vi "Ramp.vi"(8 "Control":u32, 9 "Switch 2":bool, 10 "Switch 1":bool) -> ()   [LabVIEW 2018]
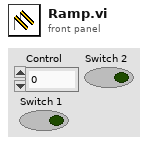
[diagram p1: front panel]
types:
  T1 = typedef "WPI_MotorControlDeviceRef.ctl" = cluster{"DeviceStatus":errorcluster, "Type":T2, "PWM":cluster{"PWM Channel":T3, "DeadBand":T4}, "CAN":cluster{"Device Number":u8, "SetOutput VI Ref":variant, "GetOutput VI Ref":variant, "Enable VI Ref":variant, "Disable VI Ref":variant, "Data":variant}, "Invert":bool, "DIO PWM":cluster{"PWM \"Enable\" Channel":T3, "DIOChannel":T5, "PWM Rate":dbl}}
  T2 = typedef "WPI_MotorControlType.ctl" = enum16{"PWM", "CAN", "DIO PWM"}
  T3 = typedef "FPGA_DIOPWMChannel.ctl" = enum8{"PWM 0", "PWM 1", "PWM 2", "PWM 3", "PWM 4", "PWM 5", "PWM 6", "PWM 7", "PWM 8", "PWM 9", "PWM MXP 0", "PWM MXP 1", "PWM MXP 2", "PWM MXP 3", "PWM MXP 4", "PWM MXP 5", "PWM MXP 6", "PWM MXP 7", "PWM MXP 8", "PWM MXP 9", "Invalid"}
  T4 = typedef "WPI_PWMDeadband.ctl" = cluster{"Name":string, "maxPositivePwm":i32, "minPositivePwm":i32, "centerPwm":i32, "maxNegativePwm":i32, "minNegativePwm":i32, "angularRange":u16}
  T5 = typedef "FPGA_DIOChannel.ctl" = enum8{"DIO 0", "DIO 1", "DIO 2", "DIO 3", "DIO 4", "DIO 5", "DIO 6", "DIO 7", "DIO 8", "DIO 9", "DIO MXP 0", "DIO MXP 1", "DIO MXP 2", "DIO MXP 3", "DIO MXP 4", "DIO MXP 5", "DIO MXP 6", "DIO MXP 7", "DIO MXP 8", "DIO MXP 9", "DIO MXP 10", "DIO MXP 11", "DIO MXP 12", "DIO MXP 13", "DIO MXP 14", "DIO MXP 15", "SPI Port CS1", "SPI Port CS2", "SPI Port CS3", "SPI Port MISO", "SPI Port MOSI", "Invalid"}
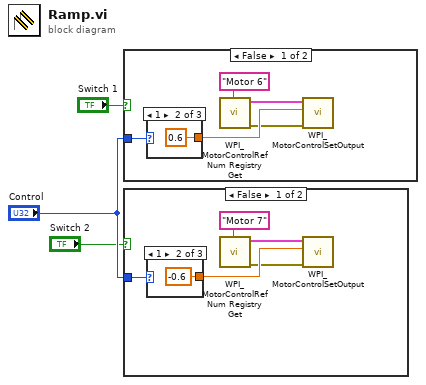
[diagram p0: block diagram]
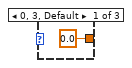
[diagram p2: hidden frame]
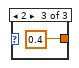
[diagram p3: hidden frame]
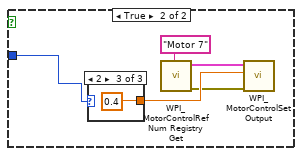
[diagram p4: hidden frame]
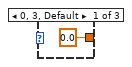
[diagram p5: hidden frame]
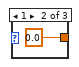
[diagram p6: hidden frame]
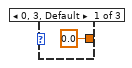
[diagram p7: hidden frame]
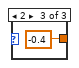
[diagram p8: hidden frame]
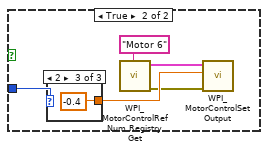
[diagram p9: hidden frame]
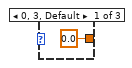
[diagram p10: hidden frame]
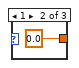
[diagram p11: hidden frame]
diagram:
  n1 = case shown="False" "Switch 1" {
    tunnel: "Control" -> [w4 w12]
    frame False {
      n2 = case shown="1" w4 {
        tunnel: [0.0 0.6 -0.4] -> w8
        frame 0, 3, Default {
        }
        frame 1 {
        }
        frame 2 {
        }
      }
      n3 = call <vilib>:"WPI_MotorControlRefNum Registry Get.vi"("refnum name"="Motor 6") -> ("error out"=w7:errorcluster, "MotorControlDevRef"=w6:T1)  [unwired: 9 in]
      n4 = call <vilib>:"WPI_MotorControlSetOutput.vi"("error in (no error)"=w7, "Output"=w8, "MotorControlDevRef"=w6) -> ()  [unwired: 6 in, 3 out]
    }
    frame True {
      n5 = case shown="2" w12 {
        tunnel: [0.0 0.0 -0.4] -> w16
        frame 0, 3, Default {
        }
        frame 1 {
        }
        frame 2 {
        }
      }
      n6 = call <vilib>:"WPI_MotorControlRefNum Registry Get.vi"("refnum name"="Motor 6") -> ("error out"=w15:errorcluster, "MotorControlDevRef"=w14:T1)  [unwired: 9 in]
      n7 = call <vilib>:"WPI_MotorControlSetOutput.vi"("error in (no error)"=w15, "Output"=w16, "MotorControlDevRef"=w14) -> ()  [unwired: 6 in, 3 out]
    }
  }
  n8 = case shown="False" "Switch 2" {
    tunnel: "Control" -> [w20 w28]
    frame False {
      n9 = case shown="1" w20 {
        tunnel: [0.0 -0.6 0.4] -> w24
        frame 0, 3, Default {
        }
        frame 1 {
        }
        frame 2 {
        }
      }
      n10 = call <vilib>:"WPI_MotorControlRefNum Registry Get.vi"("refnum name"="Motor 7") -> ("error out"=w23:errorcluster, "MotorControlDevRef"=w22:T1)  [unwired: 9 in]
      n11 = call <vilib>:"WPI_MotorControlSetOutput.vi"("error in (no error)"=w23, "Output"=w24, "MotorControlDevRef"=w22) -> ()  [unwired: 6 in, 3 out]
    }
    frame True {
      n12 = case shown="2" w28 {
        tunnel: [0.0 0.0 0.4] -> w32
        frame 0, 3, Default {
        }
        frame 1 {
        }
        frame 2 {
        }
      }
      n13 = call <vilib>:"WPI_MotorControlRefNum Registry Get.vi"("refnum name"="Motor 7") -> ("error out"=w31:errorcluster, "MotorControlDevRef"=w30:T1)  [unwired: 9 in]
      n14 = call <vilib>:"WPI_MotorControlSetOutput.vi"("error in (no error)"=w31, "Output"=w32, "MotorControlDevRef"=w30) -> ()  [unwired: 6 in, 3 out]
    }
  }
